vi "DAQmx有限数量波形数据输出.vi"() -> ()   [LabVIEW 2010]
uses:
  <vilib>/DAQmx/write.llb/DAQmx Write.vi
  <vilib>/DAQmx/write.llb/DAQmx Write (Analog 1D Wfm NChan NSamp).vi
  <vilib>/daqmx/miscellaneous.llb/DAQmx Fill In Error Info.vi
  <vilib>/measure/NI_MABase.lvlib
panel:
  in  "amplitude":dbl=1.0 format="%0.2p"
  in  "frequency":dbl=10.0 format="%0.2p"
  in  "signal type":T1(ring)
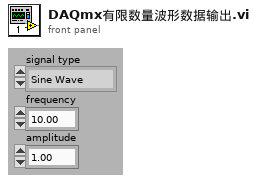
[diagram p1: front panel]
types:
  T1 = enum16{"Sine Wave", "Triangle Wave", "Square Wave", "Sawtooth Wave"}
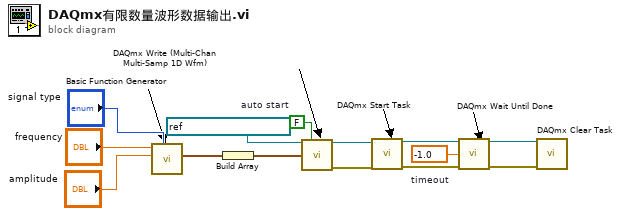
[diagram p0: block diagram]
diagram:
  w10 = -1.0  # timeout
  w14 = FALSE  # auto start
  n1 = call <vilib>:"Basic Function Generator.vi"("signal type"="signal type", "amplitude"="amplitude", "frequency"="frequency") -> ("signal out"=w5:waveform(dbl))  [unwired: 6 in, 2 out]
  n2 = Build Array(w5) -> (w4:waveform(dbl)[])
  n3 = call-poly "DAQmx Write (Multi-Chan Multi-Samp 1D Wfm).vi"("task/channels in"=refnum<k21> "我的电压输出任务", "auto start"=w14, "data"=w4) -> ("task out"=w9:refnum<k21>, "error out"=w8:errorcluster)  [unwired: 10 in, 1 out]
  n4 = call <vilib>:"DAQmx Start Task.vi"("task/channels in"=w9, "error in"=w8) -> ("task out"=w13:refnum<k21>, "error out"=w12:errorcluster)  [unwired: 12 in]
  n5 = call <vilib>:"DAQmx Wait Until Done.vi"("task/channels in"=w13, "timeout (sec)"=w10, "error in"=w12) -> ("task out"=w7:refnum<k21>, "error out"=w11:errorcluster)  [unwired: 11 in]
  n6 = call <vilib>:"DAQmx Clear Task.vi"("task in"=w7, "error in"=w11) -> ()  [unwired: 13 in, 1 out]
